vi "OPO_Align_Simulator.vi"(8 "error in (no error)":errorcluster, 11 "OPO wavelength":i32) -> (0 "error out":errorcluster, 3 "OPO Energy":dbl)   [LabVIEW 2020]
panel:
  out "Message":string
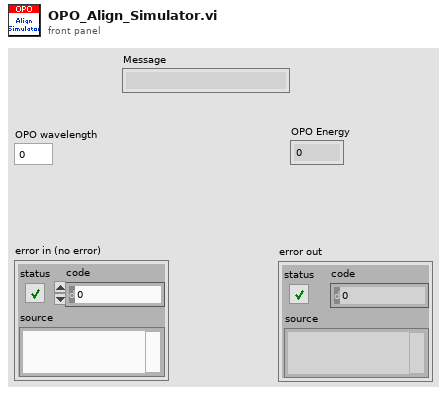
[diagram p1: front panel]
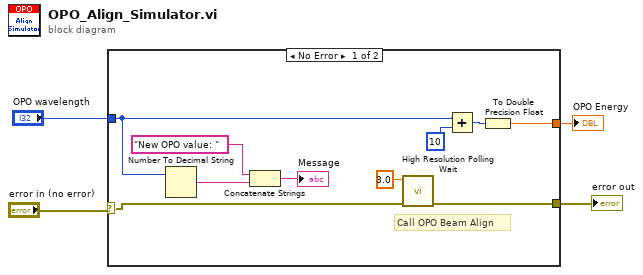
[diagram p0: block diagram]
diagram:
  n1 = case shown="No Error" "error in (no error)" {
    selector: "error in (no error)" -> [w9 w15]
    tunnel: [w8 w15] -> w3
    tunnel: "OPO wavelength" -> [w7 _]
    tunnel: [w6 _] -> w1
    frame No Error {
      # "Call OPO Beam Align"
      n2 = Number To Decimal String(number=w7) -> (decimal integer string=w13:string)  [unwired: 1 in]
      n3 = Concatenate Strings("New OPO value: " ("string"), w13) -> (→"Message":string)
      n4 = call <vilib>:"High Resolution Polling Wait.vi"("error in (no error)"=w9, "seconds to wait"=3.0) -> ("error out"=w8:errorcluster)  [unwired: 9 in]
      n5 = Add(x=w7, y=10) -> (x+y=w10:i32)
      n6 = To Double Precision Float(number=w10) -> (double precision float=w6:dbl)
    }
    frame Error {
    }
  }
  "error out" <- w3
  "OPO Energy" <- w1
